vi "phase_shifts.vi"(0 "Piezo":i32, 2 "AOTF":i32, 5 "Camera Exposure":i32) -> (11 "rangeShift":u32, 12 "mirrorL":u32, 13 "cameraR":u32, 14 "mirrorR":u32, 15 "piezoL":u32, 16 "piezoR":u32, 17 "aotfL":u32, 18 "aotfR":u32, 19 "cameraL":u32)   [LabVIEW 2013]
panel:
  out "minShift":i32
  out "maxShift":i32
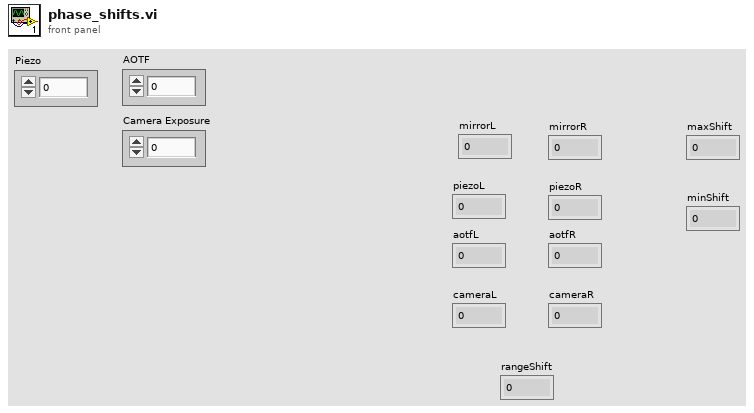
[diagram p1: front panel]
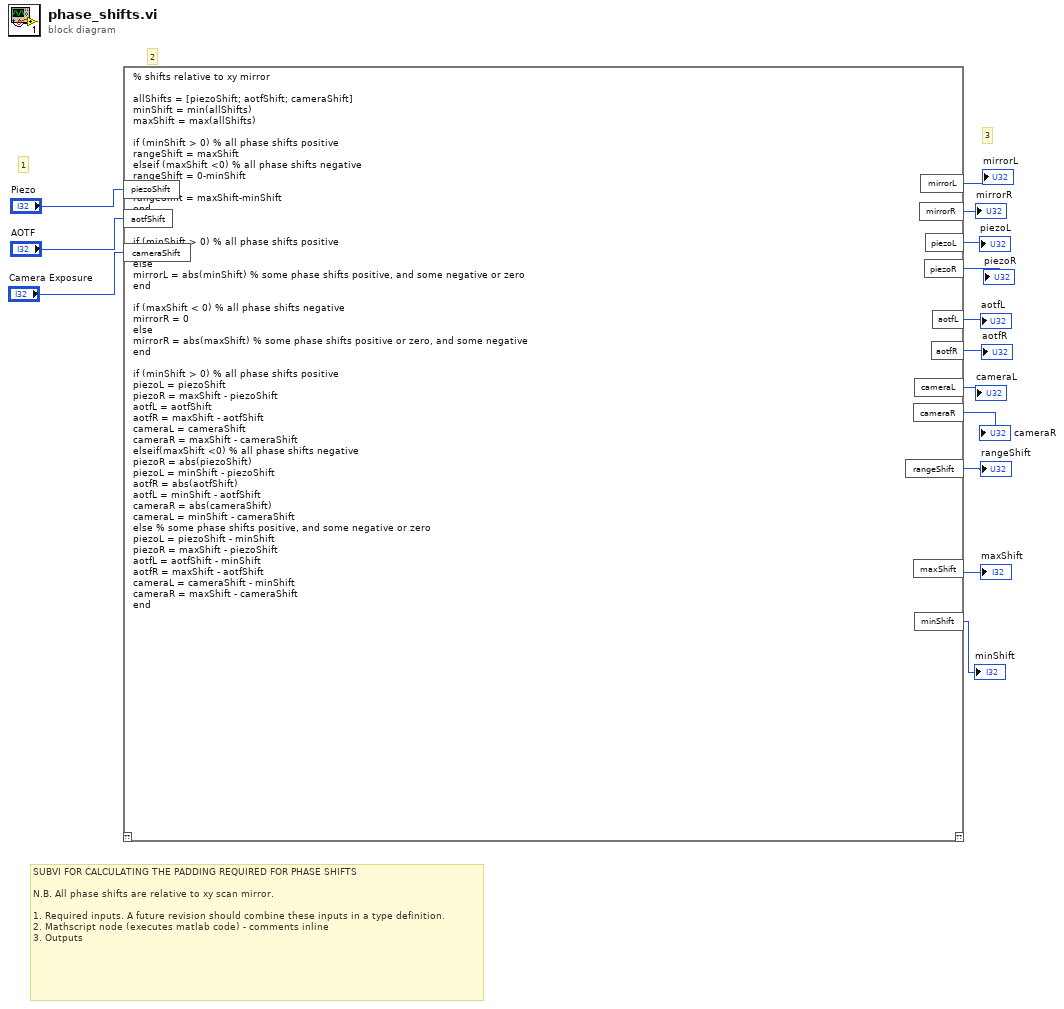
[diagram p0: block diagram]
diagram:
  # "3"
  # "2"
  # "1"
  # "SUBVI FOR CALCULATING THE PADDING REQUIRED FOR PHASE SHIFTS\n\nN.B. All phase shifts are relative to xy scan mirror.\n\n1. Required inputs. A future revision should combine these inputs in a type definition.\n2. Mathscript node (executes matlab code) - comments inline\n3. Outputs"
  n1 = mathscript code="% shifts relative to xy mirror\n\nallShifts = [piezoShift; aotfShift; cameraShift]\nminShift = min(allShifts)\nmaxShift = max(allShifts)\n\nif (minShift > 0) % all phase shifts positive\nrangeShift = maxShift\nelseif (maxShift <0) % all phase shifts negative\nrangeShift = 0-minShift\nelse\nrangeShift = maxShift-minShift\nend\n\n\nif (minShift > 0) % all phase shifts positive\nmirrorL = 0\nelse\nmirrorL = abs(minShift) % some phase shifts positive, and some negative or zero\nend\n\nif (maxShift < 0) % all phase shifts negative\nmirrorR = 0\nelse\nmirrorR = abs(maxShift) % some phase shifts positive or zero, and some negative\nend\n\nif (minShift > 0) % all phase shifts positive\npiezoL = piezoShift\npiezoR = maxShift - piezoShift\naotfL = aotfShift\naotfR = maxShift - aotfShift\ncameraL = cameraShift\ncameraR = maxShift - cameraShift\nelseif(maxShift <0) % all phase shifts negative\npiezoR = abs(piezoShift)\npiezoL = minShift - piezoShift\naotfR = abs(aotfShift)\naotfL = minShift - aotfShift\ncameraR = abs(cameraShift)\ncameraL = minShift - cameraShift\nelse % some phase shifts positive, and some negative or zero\npiezoL = piezoShift - minShift\npiezoR = maxShift - piezoShift\naotfL = aotfShift - minShift\naotfR = maxShift - aotfShift\ncameraL = cameraShift - minShift\ncameraR = maxShift - cameraShift\nend"("piezoShift"="Piezo", "aotfShift"="AOTF", "cameraShift"="Camera Exposure") -> ("mirrorL"=→"mirrorL":i32, "mirrorR"=→"mirrorR":i32, "piezoL"=→"piezoL":i32, "piezoR"=→"piezoR":i32, "cameraL"=→"cameraL":i32, "cameraR"=→"cameraR":i32, "aotfL"=→"aotfL":i32, "aotfR"=→"aotfR":i32, "rangeShift"=→"rangeShift":i32, "maxShift"=→"maxShift":i32, "minShift"=→"minShift":i32)  [unwired: 1 in, 1 out]
